vi "Test Insert Image ARGB Mask ARGB.vi"(8 "error in (no error)":errorcluster, 11 "Test Case In":refnum<class "01_Image.lvclass">) -> (0 "error out":errorcluster, 3 "Test Case Out":refnum<class "01_Image.lvclass">)   [LabVIEW 2020, in "test.lvlib" / "01_Image.lvclass"]
uses:
  01_Image.lvclass
  C:/Program Files (x86)/National Instruments/LabVIEW 2026/vi.lib/Astemes/LUnit/Test Case.lvclass
  common/Image Size (Integer).ctl
  image/ARGB Colour.ctl
  image/Line Type.ctl
  <vilib>/Astemes/LUnit/Test Case.lvclass/Test Case.ctl
  image/New Image (ARGB Preallocated).vi
  image/Draw Image to Picture (ARGB).vi
  4993e8ee-a06a-463a-9684-69129f64d5ce.vi
  image/Copy Array to Image.vi
  image/Copy Array to Image (ARGB).vi
  image/New Image (ARGB Preallocated).vi/3321fa97-f432-4e1e-8db9-a0df79aed21b.vi
  image/ARGB Colour to U32 Pixel Value.vi
  image/Draw Circle (ARGB).vi/8336a1cf-e433-4bea-8080-376bdb783d4e.vi
  image/Insert Image (ARGB with ARGB Mask).vi/5e3288c8-ee88-4cfe-89cf-31ceca475f5a.vi
  image/Draw Image to Picture (ARGB).vi/8cd07b1b-062e-4fe4-9e87-2eb3dc89fe0e.vi
  <vilib>/Astemes/LUnit/Core/LUnit Test Case/Private/Append Pass Result.vi
  <vilib>/Astemes/LUnit/Core/LUnit Test Case/Private/Append Fail Result.vi
  4993e8ee-a06a-463a-9684-69129f64d5ce.vi/9c5d11cd-9439-4240-a1ee-d9baace9c924.vi
  <vilib>/Astemes/LUnit/Core/LUnit Test Case/Private/Run In UI.vi
  <vilib>/Utility/error.llb/Clear Errors.vi
  <vilib>/Utility/error.llb/Error Cluster From Error Code.vi
  <vilib>/picture/pixmap.llb/Flatten Pixmap.vi
  image/image.lvlib
  common/common.lvlib
panel:
  out "Picture":picture
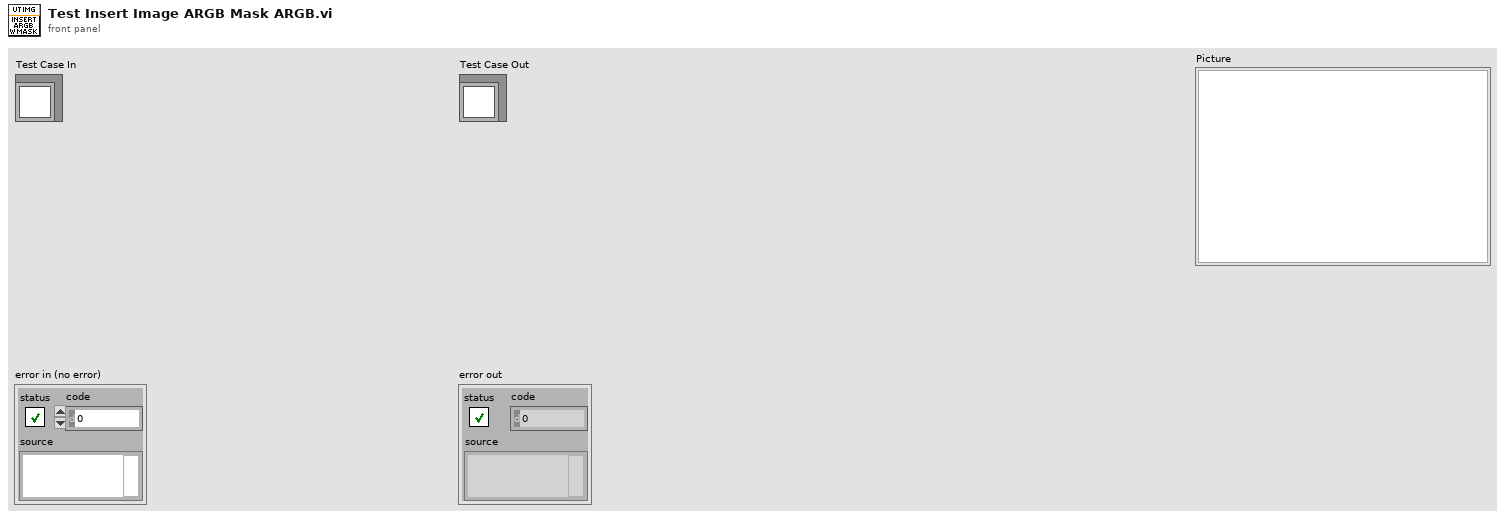
[diagram p1: front panel]
types:
  T1 = typedef "image.lvlib/Line Type.ctl" = enum8{"FILLED", "LINE_4", "LINE_8", "LINE_AA"}
  T2 = typedef "image.lvlib/ARGB Colour.ctl" = cluster{"Alpha":u8, "RGB":u32}
  T3 = typedef "common.lvlib/Image Size (Integer).ctl" = cluster{"Width":u16, "Height":u16}
  T4 = typedef "image.lvlib/ARGB Image.ctl" = refnum<data-value>
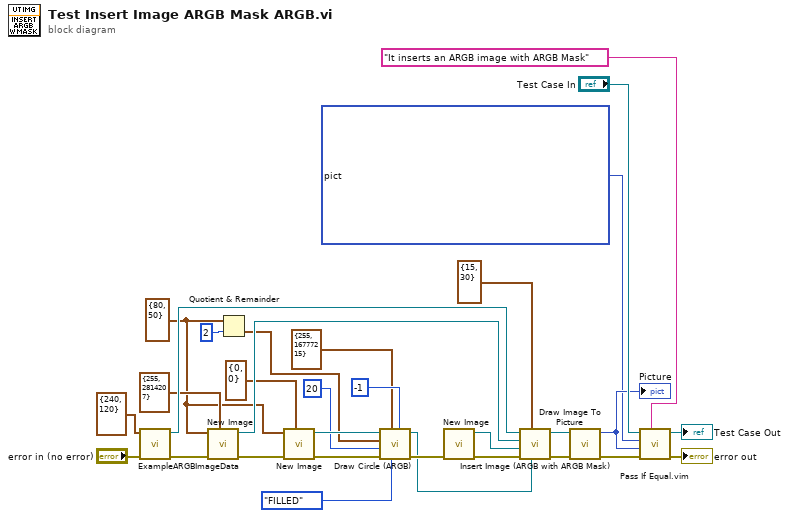
[diagram p0: block diagram]
diagram:
  w11 = T3 {"Width"=80, "Height"=50} ("Preallocated Image Size")
  n1 = call "ExampleARGBImageData.vi"("error in (no error)"="error in (no error)", "Image Size"=T3 {"Width"=240, "Height"=120} ("Preallocated Image Size (Default - 0,0)")) -> ("error out"=w20:errorcluster, "Data Value Reference out"=w25:T4)  [unwired: 6 in, 2 out]
  n2 = call-poly "New Image.vi"("Colour (Default: Black)"=T2 {"Alpha"=255, "RGB"=2814207}, "error in (no error)"=w20, "Preallocated Image Size (Default: 0,0)"=w11) -> ("error out"=w17:errorcluster, "ARGB Image"=w19:T4)  [unwired: 7 in]
  n3 = Quotient & Remainder(x=w11, y=u16 2) -> (floor(x/y)=w9:T3)  [unwired: 1 out]
  n4 = call-poly "New Image.vi"("Colour (Default: Black)"=T2 {"Alpha"=0, "RGB"=0}, "error in (no error)"=w17, "Preallocated Image Size (Default: 0,0)"=w11) -> ("error out"=w16:errorcluster, "ARGB Image"=w15:T4)  [unwired: 7 in]
  n5 = call "Draw Circle (ARGB).vi"("Thickness (Default: 1)"=-1, "OpenCV Line Type (Default LINE_8)"=Line_Type."FILLED", "ARGB Colour"=T2 {"Alpha"=255, "RGB"=16777215}, "error in (no error)"=w16, "Radius"=u16 20, "Centre"=w9, "ARGB Image in"=w15) -> ("error out"=w14:errorcluster, "ARGB Image"=w13:T4)  [unwired: 3 in]
  n6 = call-poly "New Image.vi"("error in (no error)"=w14) -> ("error out"=w27:errorcluster, "ARGB Image"=w22:T4)  [unwired: 9 in]
  n7 = call "Insert Image (ARGB with ARGB Mask).vi"("ARGB Image Mask in"=w13, "Offset (Default: 0,0)"=T3 {"Width"=15, "Height"=30}, "error in (no error)"=w27, "ARGB Image Destination in"=w22, "ARGB Image Child in"=w19, "ARGB Image Parent in"=w25) -> ("error out"=w7:errorcluster, "ARGB Image Destination"=w21:T4)  [unwired: 4 in]
  n8 = call-poly "Draw Image To Picture.vi"("error in (no error)"=w7, "ARGB Image Source in"=w21) -> ("error out"=w6:errorcluster, "Picture"=w5:picture)  [unwired: 8 in]
  "Picture" <- w5
  n9 = call "Pass If Equal.vim"("Description"="It inserts an ARGB image with ARGB Mask", "error in (no error)"=w6, "Actual"=w5, "Expected"=picture bytes[86430] ("Picture"), "LUnit Test Case In"="Test Case In") -> ("error out"=→"error out":errorcluster, "LUnit Test Case Out"=→"Test Case Out":refnum<class "01_Image.lvclass">)  [unwired: 5 in]
